vi "Write WaveformQueues.vi"(8 "error in (no error)":errorcluster, 10 "WaveformQueues":T1, 11 "Generator in":refnum<class "Generator.lvclass">) -> (0 "error out":errorcluster, 3 "Generator out":refnum<class "Generator.lvclass">)   [LabVIEW 2019, in "Generator.lvclass"]
uses:
  Generator.lvclass
  typedefs/WaveformQueues--Cluster.ctl
  Generator.lvclass/Generator.ctl
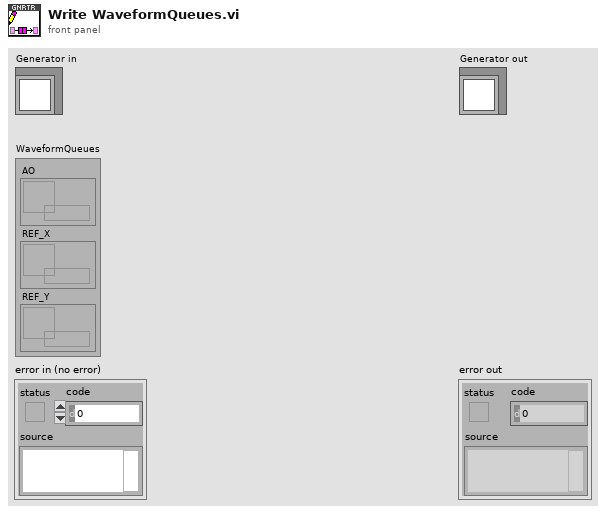
[diagram p1: front panel]
types:
  T1 = typedef "Generator.lvclass/WaveformQueues--Cluster.ctl" = cluster{"AO":refnum<queue>, "REF_X":refnum<queue>, "REF_Y":refnum<queue>}
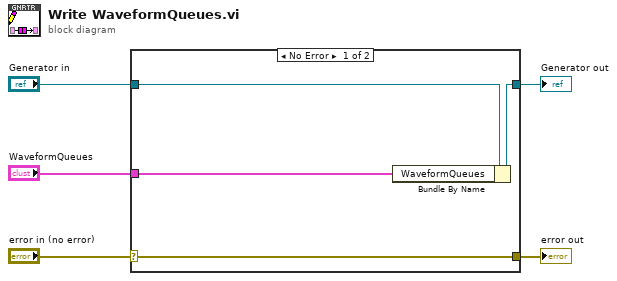
[diagram p0: block diagram]
diagram:
  n1 = case shown="No Error" "error in (no error)" {
    selector: "error in (no error)" -> [w9 w10]
    tunnel: [w9 w10] -> w4
    tunnel: [w7 w11] -> w2
    tunnel: "Generator in" -> [w8 w11]
    tunnel: "WaveformQueues" -> [w6 _]
    frame No Error {
      n2 = Bundle By Name(cluster=w8, "WaveformQueues"=w6) -> (w7:refnum<class "Generator.lvclass">)
    }
    frame Error {
    }
  }
  "error out" <- w4
  "Generator out" <- w2
